vi "Autotuning PID Closed Loop Step.vi"() -> ()   [LabVIEW 2019]
doc: "This example demonstrates how to use the PID Design function to obtain PID parameters based on measured process."
uses:
  <vilib>/Rock Robotics/WPI/ThirdParty/JAS_Junk/TrajLib/PIDController_AtSetpoint.vi
  <vilib>/Rock Robotics/WPI/ThirdParty/JAS_Junk/TrajLib/PIDController_SetPIDF.vi
  <vilib>/Rock Robotics/WPI/ThirdParty/JAS_Junk/TrajLib/PIDController_SetDerivativeFilter.vi
  <vilib>/Rock Robotics/WPI/ThirdParty/JAS_Junk/TrajLib/PIDController_SetIntegratorRange.vi
  <vilib>/Rock Robotics/WPI/ThirdParty/JAS_Junk/TrajLib/PIDController_SetTolerancePandV.vi
  <vilib>/Rock Robotics/WPI/ThirdParty/JAS_Junk/TrajLib/PIDController_DisableContinousInput.vi
  <vilib>/Rock Robotics/WPI/ThirdParty/JAS_Junk/TrajLib/PIDController_EnableContinousInput.vi
  <vilib>/Rock Robotics/WPI/ThirdParty/JAS_Junk/TrajLib/PIDController_Reset.vi
  <vilib>/Rock Robotics/WPI/ThirdParty/JAS_Junk/TrajLib/PIDController_New.vi
  <vilib>/Rock Robotics/WPI/ThirdParty/JAS_Junk/TrajLib/PIDController_SetOutputLimits.vi
  <vilib>/Rock Robotics/WPI/ThirdParty/JAS_Junk/TrajLib/PIDController_NewPeriod.vi
  <vilib>/Rock Robotics/SystemInterfaces/NetworkCommunication/NetComm_UsageReport_report.vi
  <vilib>/Rock Robotics/WPI/ThirdParty/JAS_Junk/TrajLib/Util_LibraryGlobals.vi
  <vilib>/Rock Robotics/WPI/ThirdParty/JAS_Junk/TrajLib/PIDController_AdvCalculate_FF_Sp_Pv.vi
  <vilib>/Rock Robotics/WPI/ThirdParty/JAS_Junk/TrajLib/Trajectory_Library.lvlib
panel:
  in  "Controller Constant Type":T1(ring)=enum."Ziegler Nicols - Normal"
  out "Error Occured":bool
  out "Elapsed Time":dbl format="%13.2f"
  in  "MinimumIntegral":dbl=-100.0 format="%#_13g"
  in  "MaximumIntegral":dbl=100.0 format="%#_13g"
  in  "Kn":dbl=0.4 format="%#_13g"
  in  "Use\nFeedforward":bool
  out "Tuned PID Gains":T2
  in  "CO Step Offset":dbl=2.0 format="%#_13g"
  out "Tuning Complete":bool
  in  "Type of controller":u16(ring)=2 items=["P", "PI", "PID"]
  in  "Tab Control":T3(tab)
  in  "Instructions":string="Overview: This example demonstrates how to use the PID Autotuning Design to obtain PID parameters based on setpoint and process variable collected in another loop.\nInstructions:\n1. Run the VI and wait until the process variable (PV) reaches near setpoint (SP).\n2.  In the PID Autotuning Design section, select the type of algorithm, type of controller and excitation amplitude for the 'open loop step response'. Then, click Autotune to start the process. Select the Identified Plant Parameter tab and see the results from the identification.\n3.  When the tuned PID gains do not change anymore, the identification is done and you have the option to accept by clicking Accept gain, which will transfer the new gain to PID Gains.\n4. Click the Autotune button again to go back to the automatic control state. You can try different options and repeat this process.\n5. Click Stop to stop the VI.\n"
  out "Plant and Test Data":T4
  in  "Process parameters":T5={"static gain"=2.5, "lag (s)"=2.5, "deadtime (s)"=0.01, "load"=0.0, "deadband"=0.0, "sensor noise"=0.005, "initial PV"=30.0, "plant noise"=0.005}
  out "Diagnostic":T6
  in  "PID \nAuto / Manual":bool=TRUE
  out "CO Chart":dbl(graph)=20.39115328927357
  in  "Accept gain":bool
  in  "Perform PID\nAutoTune":bool
  in  "SP:":dbl(slide)=50.98039215686275 min=0.0 max=0.0 scale=0.0..100.0
  out "CO_":dbl(slide)=20.39115328927357 scale=-100.0..100.0
  out "PV:":dbl(slide)=50.98160323470328 scale=0.0..100.0
  in  "PID Gains":T7={"proportional gain (Kp)"=2.5, "integral time (Ki, /sec)"=4.0, "derivative time (Kd, /sec)"=0.0} {"derivative time (Kd, /sec)" format="%#.6g"; "integral time (Ki, /sec)" format="%#.6g"; "proportional gain (Kp)" format="%#.6g"}
  in  "Sampling Time dt (s)":dbl=0.019999999999999997 min=0.001 step=0.01 format="%#.3p"
  out "SP and PV":cluster{"initial PV":dbl, "SP1:":dbl}(graph)={"initial PV"=50.98160323470328, "SP1:"=50.98039215686275}
  # "Proportional-Integral-Derivative (PID) Controller"
  # "PID Autotuning Design"
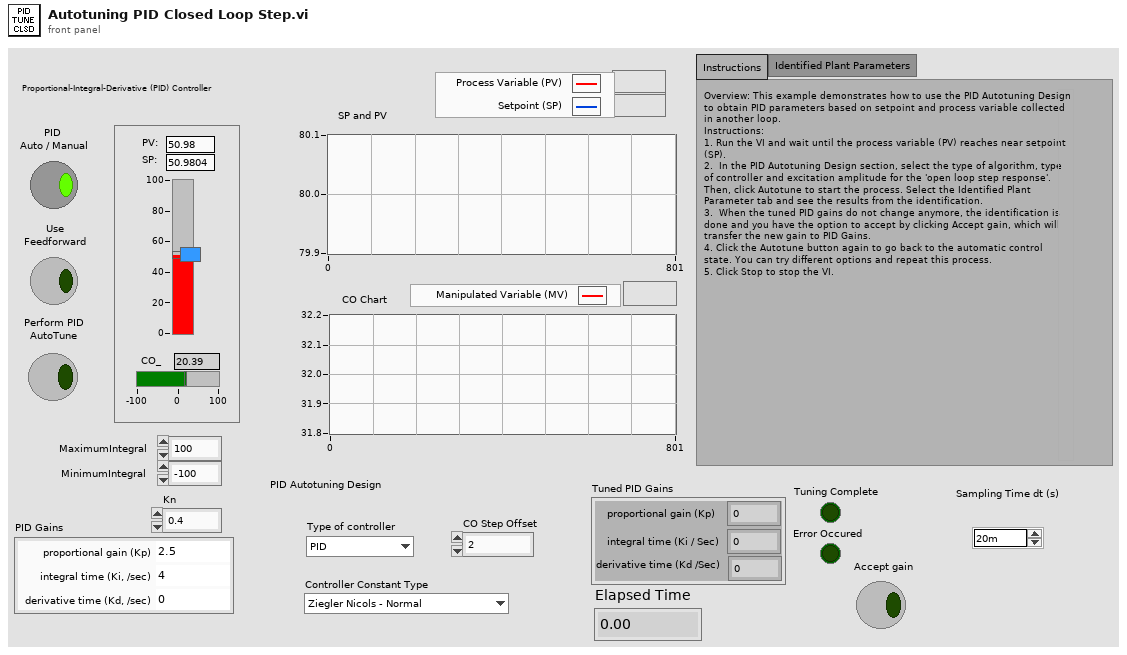
[diagram p1: front panel]
types:
  T1 = enum16{"Ziegler Nicols - Fast", "Ziegler Nicols - Normal", "Ziegler Nicols - Slow", "CHR regulator - 0% overshoot", "CHR regulator - 20% overshoot", "CHR servo - 0 % overshoot", "CHR servo - 20% overshoot"}
  T2 = cluster{"proportional gain (Kp)":dbl, "integral time (Ki / Sec)":dbl, "derivative time (Kd /Sec)":dbl}
  T3 = enum32{"Instructions", "Identified Plant Parameters"}
  T4 = cluster{"Plant Gain (K)":dbl, "Time Constant (T)":dbl, "Dead Time (L)":dbl, "stimulus operating point":dbl, "response operating point":dbl}
  T5 = cluster{"static gain":dbl, "lag (s)":dbl, "deadtime (s)":dbl, "load":dbl, "deadband":dbl, "sensor noise":dbl, "initial PV":dbl, "plant noise":dbl}
  T6 = cluster{"Const Done":bool, "Plant Done":bool, "PV Std Dev":dbl, "CO Std Dev":dbl}
  T7 = cluster{"proportional gain (Kp)":dbl, "integral time (Ki, /sec)":dbl, "derivative time (Kd, /sec)":dbl}
  T8 = typedef "Trajectory_Library.lvlib/PID_ADV_LIMITS.ctl" = cluster{"MaxInput":dbl, "MinInput":dbl, "Continuous":bool, "MaxOutput":dbl, "MinOutput":dbl}
  T9 = typedef "Trajectory_Library.lvlib/PID_ADV_TUNING.ctl" = cluster{"Kf":dbl, "Kp":dbl, "Ki":dbl, "Kd":dbl, "MaximumIntegral":dbl, "MinimumIntegral":dbl, "Filter Derivative":bool}
  T10 = cluster{"Controller Constant Type":enum16{"Ziegler Nicols - Fast", "Ziegler Nicols - Normal", "Ziegler Nicols - Slow", "CHR regulator - 0% overshoot", "CHR regulator - 20% overshoot", "CHR servo - 0 % overshoot", "CHR servo - 20% overshoot"}, "Type of Controller":enum16{"P", "PI", "PID"}, "CO Offset":dbl, "Kn":dbl, "Tuning Tolerance":dbl, "Plant Tolerance":dbl, "Newest Avg Time ":i32, "Long Ave Time":i32}
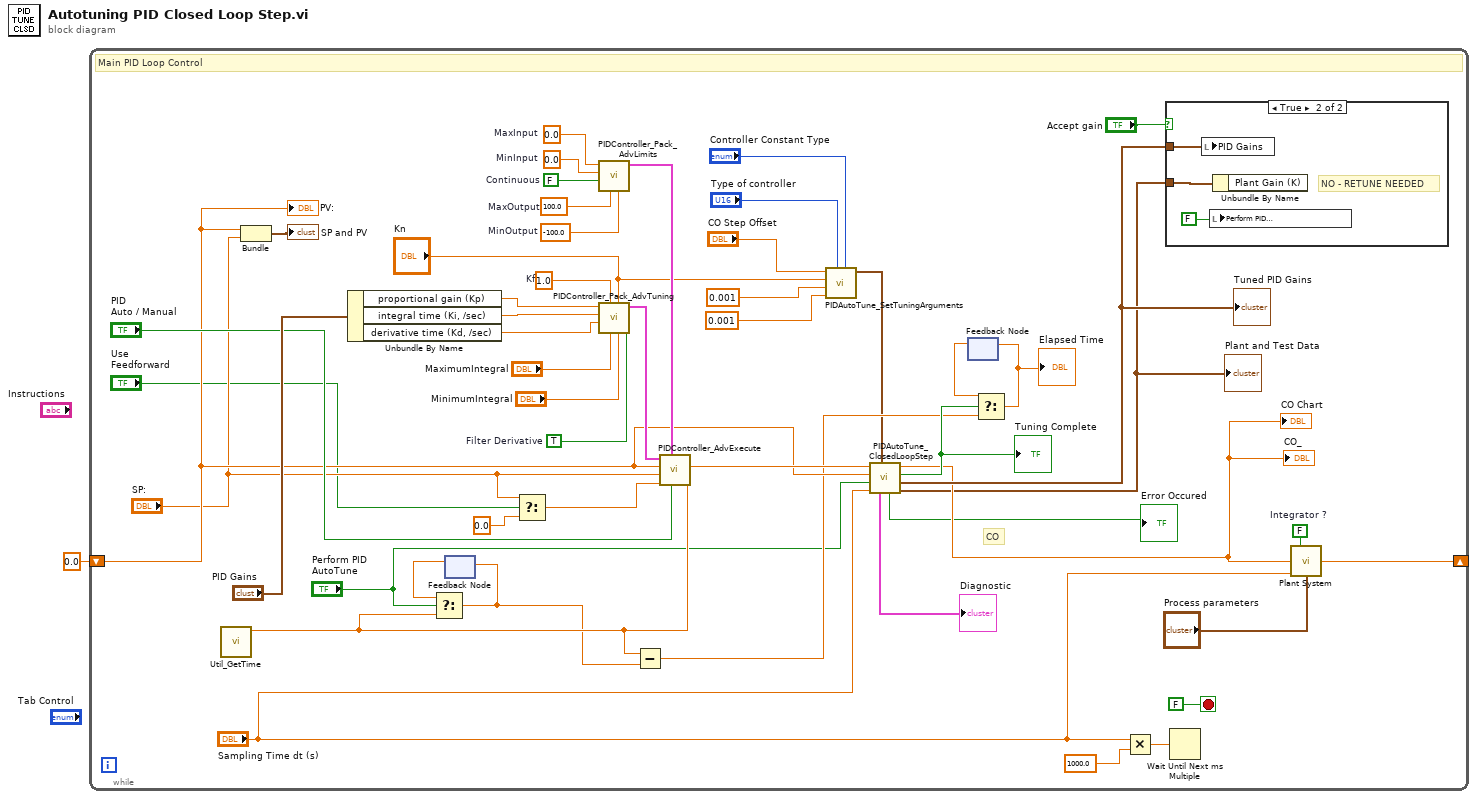
[diagram p0: block diagram]
diagram:
  n1 = while {
    shift-left: 0.0 ("Plant Output") -> [w29]
    shift-right: [w50] -> _
    stop <- FALSE stop-if-true
    w46 = 1.0  # Kf
    w43 = TRUE  # Filter Derivative
    w41 = 0.0  # MinInput
    w40 = FALSE  # Continuous
    w39 = 100.0  # MaxOutput
    w42 = -100.0  # MinOutput
    w38 = 0.0  # MaxInput
    w51 = FALSE  # Integrator ?
    # "CO"
    # "Main PID Loop Control"
    n2 = call <vilib>:"Util_GetTime.vi"() -> ("FPGA_Time_Seconds"=w25:dbl)  [unwired: 10 in, 1 out]
    n3 = Bundle("Plant Output"=w29, "SP:"="SP:") -> (→"SP and PV":cluster{"Plant Output":dbl, "SP:":dbl})  [unwired: 1 in]
    n4 = Unbundle By Name("PID Gains") -> ("proportional gain (Kp)"=w34:dbl, "integral time (Ki, /sec)"=w33:dbl, "derivative time (Kd, /sec)"=w32:dbl)
    n5 = feedback #1() -> (w26:dbl)  [unwired: 1 in]
    n6 = Select(t=w26, s="Perform PID\nAutoTune", f=w25) -> (s? t:f=w24:dbl)
    n7 = feedback-in #1(w24) -> ()
    n8 = Select(t="SP:", s="Use\nFeedforward", f=0.0) -> (s? t:f=w16:dbl)
    n9 = call <vilib>:"PIDController_Pack_AdvLimits.vi"("MinOutput"=w42, "MaxOutput"=w39, "Continuous"=w40, "MinInput"=w41, "MaxInput"=w38) -> ("Adv PID Limits"=w36:T8)  [unwired: 6 in]
    n10 = call <vilib>:"PIDController_Pack_AdvTuning.vi"("Filter Derivative"=w43, "MinimumIntegral"="MinimumIntegral", "Kn"="Kn", "MaximumIntegral"="MaximumIntegral", "Kf"=w46, "Kd"=w32, "Ki"=w33, "Kp"=w34) -> ("Adv PID Tuning"=w37:T9)  [unwired: 3 in]
    n11 = Subtract(x=w25, y=w24) -> (x-y=w22:dbl)
    n12 = call <vilib>:"PIDController_AdvExecute.vi"("Time"=w25, "Auto"="PID \nAuto / Manual", "Adv PID Limits"=w36, "FF-FeedForward"=w16, "SP-SetPoint"="SP:", "PV-Measurement"=w29, "Adv PID Tuning"=w37) -> ("CO-ControlOutput"=w30:dbl)  [unwired: 2 in, 2 out]
    n13 = call <vilib>:"PIDAutoTune_SetTuningArguments.vi"("Controller Constant Type"="Controller Constant Type", "Type of Controller"="Type of controller", "Plant Tolerance"=0.001, "Tuning Tolerance"=0.001, "Kn"="Kn", "CO Offset"="CO Step Offset") -> ("Configuration Parameters"=w2:T10)  [unwired: 5 in]
    n14 = call <vilib>:"PIDAutoTune_ClosedLoopStep.vi"("Configuration Parameters"=w2, "Sampling Time dt (s)"="Sampling Time dt (s)", "Tune"="Perform PID\nAutoTune", "Measurement  (PV)"=w29, "Control Output (Co)"=w30) -> ("Plant and Test Data"=w13:T4, "New Tuning Parameters"=w27:T2, "Tuning Done"=w23:bool, "Adj CO"=w18:dbl, "Error Occured"=→"Error Occured":bool, "Diagnostic"=→"Diagnostic":T6)  [unwired: 1 in]
    "CO Chart" <- w18
    "CO_" <- w18
    "Tuning Complete" <- w23
    "Plant and Test Data" <- w13
    "Tuned PID Gains" <- w27
    n15 = feedback #2() -> (w20:dbl)  [unwired: 1 in]
    n16 = Select(t=w20, s=w23, f=w22) -> (s? t:f=w21:dbl)
    "Elapsed Time" <- w21
    n17 = feedback-in #2(w21) -> ()
    n18 = Multiply(x="Sampling Time dt (s)", y=1000.0) -> (x*y=w48:dbl)
    n19 = case shown="True" "Accept gain" {
      tunnel: w27 -> [_ w55]
      tunnel: w13 -> [_ w53]
      frame False {
      }
      frame True {
        # "NO - RETUNE NEEDED"
        n20 = local write "PID Gains"(w55) -> ()
        n21 = local write "Perform PID\nAutoTune"(FALSE ("Autotune")) -> ()
        n22 = Unbundle By Name(w53) -> ()  [unwired: 1 out]
      }
    }
    n23 = Wait Until Next ms Multiple(millisecond multiple=w48) -> ()  [unwired: 1 out]
    n24 = call "Plant System.vi"("Integrator ?"=w51, "Plant Input"=w18, "dt (s)"="Sampling Time dt (s)", "process parameters"="Process parameters") -> ("Plant Output"=w50:dbl)  [unwired: 11 in]
    "PV:" <- w29
  }
